vi "Excercise 3-7.vi"() -> ()   [LabVIEW 2014]
panel:
  out "Square Root Value":dbl
  in  "Number":dbl
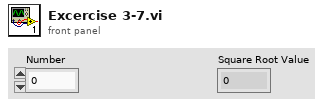
[diagram p1: front panel]
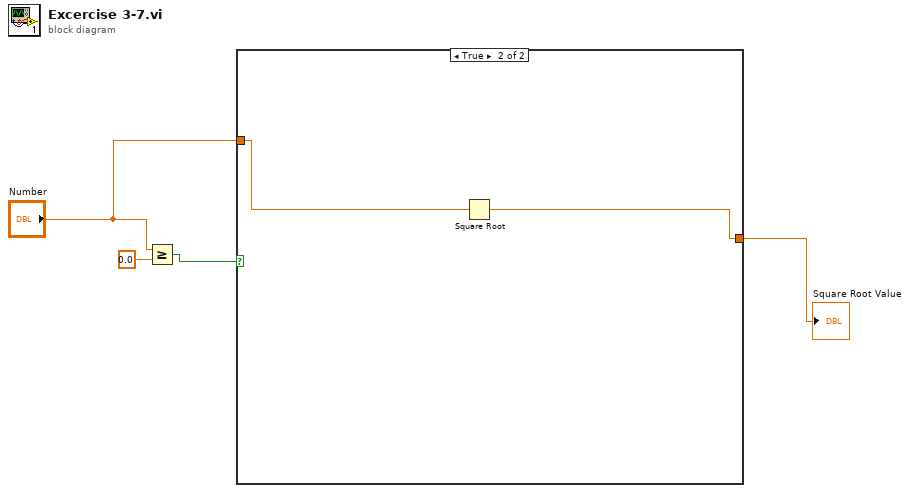
[diagram p0: block diagram]
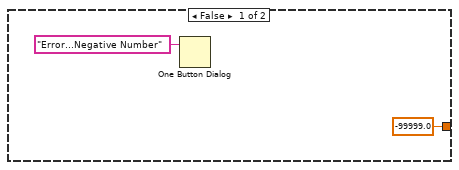
[diagram p2: hidden frame]
diagram:
  n1 = Greater Or Equal?(x="Number", y=0.0) -> (x >= y?=w3:bool)
  n2 = case shown="True" w3 {
    tunnel: "Number" -> [_ w8]
    tunnel: [-99999.0 ("Number") w7] -> w1
    frame False {
      n3 = One Button Dialog(message="Error...Negative Number") -> ()  [unwired: 1 in, 1 out]
    }
    frame True {
      n4 = Square Root(x=w8) -> (sqrt(x)=w7:dbl)
    }
  }
  "Square Root Value" <- w1
